vi "solar_excel Worksheet Format (Range).vi"(6 "Format":T1, 8 "error in (no error)":errorcluster, 9 "End (1,1 = 'A1')":cluster{"Row":u32, "Column":u32}, 10 "Start (1,1 = 'A1')":cluster{"Row":u32, "Column":u32}, 11 "Excel Worksheet in":T2) -> (0 "error out":errorcluster, 3 "Excel Worksheet out":T2)   [LabVIEW 2018]
doc: "This formats a range of cells."
uses:
  solar_excel_ctl Worksheet.ctl
  solar_excel_ctl TSV.ctl
  solar_excel_ctl Format.ctl
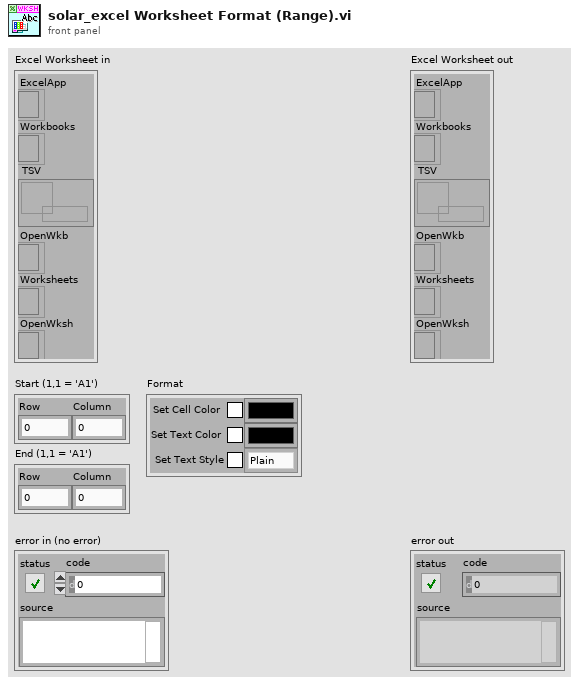
[diagram p1: front panel]
types:
  T1 = typedef "solar_excel_ctl Format.ctl" = cluster{"Set Cell Color":bool, "Cell Color":u32, "Set Text Color":bool, "Text Color":u32, "Set Text Style":bool, "Text Style":enum8{"Plain", "Bold", "Italic"}}
  T2 = typedef "solar_excel_ctl Worksheet.ctl" = cluster{"ExcelApp":refnum<k7>, "Workbooks":refnum<k7>, "TSV":refnum<queue>, "OpenWkb":refnum<k7>, "Worksheets":refnum<k7>, "OpenWksh":refnum<k7>}
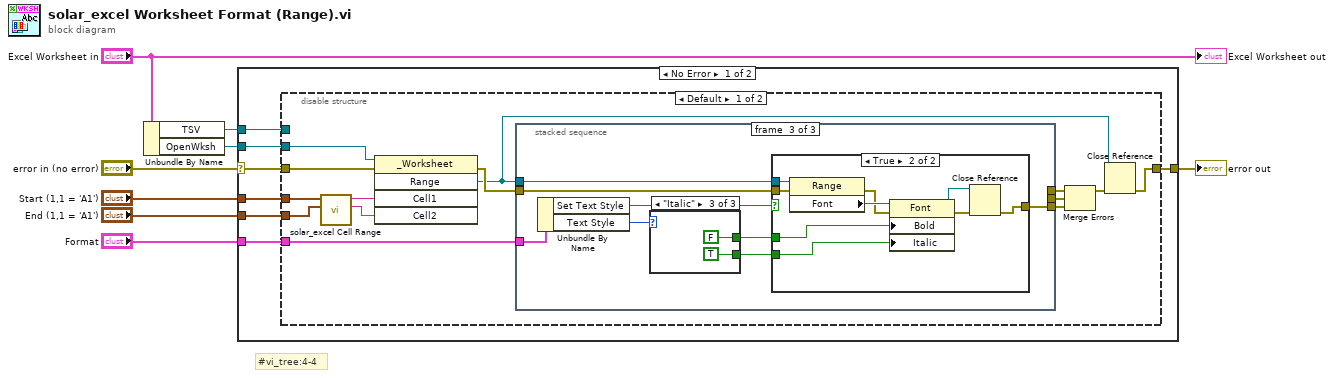
[diagram p0: block diagram]
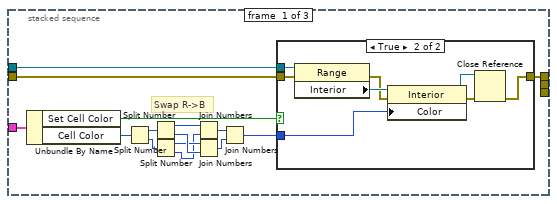
[diagram p2: hidden frame]
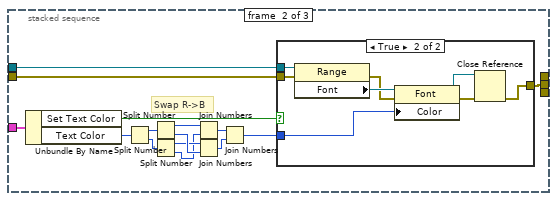
[diagram p4: hidden frame]
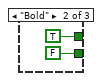
[diagram p7: hidden frame]
diagram:
  # "#vi_tree:4-4"
  n1 = Unbundle By Name("Excel Worksheet in") -> ("TSV"=w2:refnum<queue>, "OpenWksh"=w6:refnum<k7>)
  n2 = case shown="No Error" "error in (no error)" {
    selector: "error in (no error)" -> [w15 w101]
    tunnel: [w13 w101] -> w8
    tunnel: w6 -> [w14 _]
    tunnel: "Start (1,1 = 'A1')" -> [w12 _]
    tunnel: "End (1,1 = 'A1')" -> [w11 _]
    tunnel: w2 -> [w10 _]
    tunnel: "Format" -> [w9 _]
    frame No Error {
      n3 = disable-structure shown="Default" {
        disable-tunnel: w15 -> [w29 w100]
        disable-tunnel: w14 -> [w28 _]
        disable-tunnel: [w22 w100] -> w13
        disable-tunnel: w12 -> [w26 _]
        disable-tunnel: w11 -> [w25 _]
        disable-tunnel: w10 -> [_ _]
        disable-tunnel: w9 -> [w21 _]
        frame condition #0 (active) {
          n4 = call "solar_excel Cell Range.vi"("End (1,1 = 'A1')"=w25, "Start (1,1 = 'A1')"=w26) -> ("End Cell"=w23:string, "Start Cell"=w24:string)  [unwired: 7 in, 1 out]
          n5 = invoke class="_Worksheet" method="Range"(reference=w28, error in=w29, "Cell1"=w24, "Cell2"=w23) -> (error out=w27:errorcluster, "Range"=w17:refnum<k7>)  [unwired: 1 in, 3 out]
          n6 = stacked-sequence {
            tunnel: w17 -> [w44 w68 w85]
            tunnel: w27 -> [w43 w67 w84]
            tunnel: w21 -> [w42 w66 w83]
            tunnel: [w30 _ _] -> w20
            tunnel: [_ w54 _] -> w19
            tunnel: [_ _ w81] -> w16
            frame #0 {
              # "Swap R->B"
              n7 = Unbundle By Name(w42) -> ("Set Cell Color"=w31:bool, "Cell Color"=w33:u32)
              n8 = Split Number(x=w33) -> (hi(x)=w37:u16, lo(x)=w36:u16)
              n9 = Split Number(x=w37) -> (hi(x)=w41:u8, lo(x)=w40:u8)
              n10 = Split Number(x=w36) -> (hi(x)=w39:u8, lo(x)=w38:u8)
              n11 = Join Numbers(hi=w41, lo=w38) -> ((hi.lo)=w34:u16)
              n12 = Join Numbers(hi=w39, lo=w40) -> ((hi.lo)=w35:u16)
              n13 = Join Numbers(hi=w34, lo=w35) -> ((hi.lo)=w32:u32)
              n14 = case shown="True" w31 {
                tunnel: w44 -> [_ w53]
                tunnel: w43 -> [w45 w52]
                tunnel: [w45 w47] -> w30
                tunnel: w32 -> [_ w46]
                frame False {
                }
                frame True {
                  n15 = property class="Range"(reference=w53, error in=w52) -> (error out=w48:errorcluster, "Interior"=w51:refnum<k7>)  [unwired: 1 out]
                  n16 = property class="Interior"(reference=w51, error in=w48, "Color"=w46) -> (reference out=w49:refnum<k7>, error out=w50:errorcluster)
                  n17 = Close Reference(reference=w49, error in (no error)=w50) -> (error out=w47:errorcluster)
                }
              }
            }
            frame #1 {
              # "Swap R->B"
              n18 = Unbundle By Name(w66) -> ("Set Text Color"=w55:bool, "Text Color"=w57:u32)
              n19 = Split Number(x=w57) -> (hi(x)=w61:u16, lo(x)=w60:u16)
              n20 = Split Number(x=w61) -> (hi(x)=w65:u8, lo(x)=w64:u8)
              n21 = Split Number(x=w60) -> (hi(x)=w63:u8, lo(x)=w62:u8)
              n22 = Join Numbers(hi=w65, lo=w62) -> ((hi.lo)=w58:u16)
              n23 = Join Numbers(hi=w63, lo=w64) -> ((hi.lo)=w59:u16)
              n24 = Join Numbers(hi=w58, lo=w59) -> ((hi.lo)=w56:u32)
              n25 = case shown="True" w55 {
                tunnel: w68 -> [_ w77]
                tunnel: w67 -> [w69 w76]
                tunnel: [w69 w71] -> w54
                tunnel: w56 -> [_ w70]
                frame False {
                }
                frame True {
                  n26 = property class="Range"(reference=w77, error in=w76) -> (error out=w72:errorcluster, "Font"=w75:refnum<k7>)  [unwired: 1 out]
                  n27 = property class="Font"(reference=w75, error in=w72, "Color"=w70) -> (reference out=w73:refnum<k7>, error out=w74:errorcluster)
                  n28 = Close Reference(reference=w73, error in (no error)=w74) -> (error out=w71:errorcluster)
                }
              }
            }
            frame #2 {
              n29 = Unbundle By Name(w83) -> ("Set Text Style"=w82:bool, "Text Style"=w80:enum8{"Plain", "Bold", "Italic"})
              n30 = case shown="\"Italic\"" w80 {
                tunnel: [_ TRUE FALSE] -> w79
                tunnel: [_ FALSE TRUE] -> w78
                frame "Plain" {
                }
                frame "Bold" {
                }
                frame "Italic" {
                }
              }
              n31 = case shown="True" w82 {
                tunnel: w85 -> [_ w99]
                tunnel: w84 -> [w90 w98]
                tunnel: [w90 w93] -> w81
                tunnel: w79 -> [_ w92]
                tunnel: w78 -> [_ w91]
                frame False {
                }
                frame True {
                  n32 = property class="Range"(reference=w99, error in=w98) -> (error out=w94:errorcluster, "Font"=w97:refnum<k7>)  [unwired: 1 out]
                  n33 = property class="Font"(reference=w97, error in=w94, "Bold"=w92, "Italic"=w91) -> (reference out=w95:refnum<k7>, error out=w96:errorcluster)
                  n34 = Close Reference(reference=w95, error in (no error)=w96) -> (error out=w93:errorcluster)
                }
              }
            }
          }
          n35 = Merge Errors(w20, w19, w16) -> (w18:errorcluster)
          n36 = Close Reference(reference=w17, error in (no error)=w18) -> (error out=w22:errorcluster)
        }
        frame condition #1 {
          # "Do nothing"
        }
      }
    }
    frame Error {
    }
  }
  "error out" <- w8
  "Excel Worksheet out" <- "Excel Worksheet in"
